vi "QFileDialog.vi"(5 "parent":refnum<class "QWidget.lvclass">, 6 "filter":string, 8 "Error In":errorcluster, 9 "directory":string, 10 "caption":string, 11 "Post-Bundled Subclass":refnum<class "QFileDialog.lvclass">) -> (0 "Error Out":errorcluster, 3 "New QFileDialog":refnum<class "QFileDialog.lvclass">)   [LabVIEW 2014, in "QFileDialog.lvclass"]
doc: "LabVIEW-specific documentation is not yet available. See <b>http://doc.qt.io/qt-5/QFileDialog.html#QFileDialog</b>"
uses:
  QFileDialog.lvclass
  QWidget/QWidget.lvclass
  LQ Core/LQCoreEngine/_Internal/LQIdentity Registry Action.ctl
  LQ Core/LQIdentity/LQIdentity.lvclass/LQIdentity.ctl
  LQ Core/LQCoreEngine/LQCoreEngine.lvclass
  LQ Core/LQ Core.lvlib
  LQ Core/LQIdentity/LQIdentity.lvclass
panel:
  # "Copyright (c) 2016 Sze Howe Koh\n\nThis Source Code Form is subject to the terms of the Mozilla Public\nLicense, v. 2.0. If a copy of the MPL was not distributed with this\nfile, You can obtain one at http://mozilla.org/MPL/2.0/."
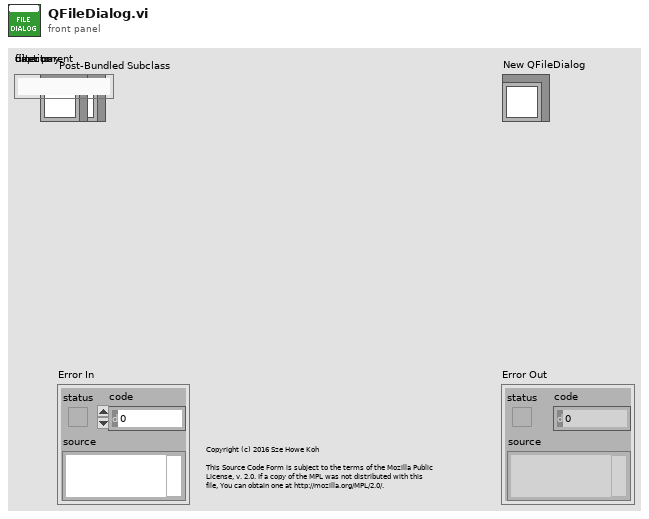
[diagram p1: front panel]
types:
  T1 = typedef "LQ Core.lvlib/LQCoreEngine.lvclass/LQIdentity Registry Action.ctl" = enum16{"Init", "Register LQIdentity", "Get LQIdentity Info", "Deregister LQIdentity"}
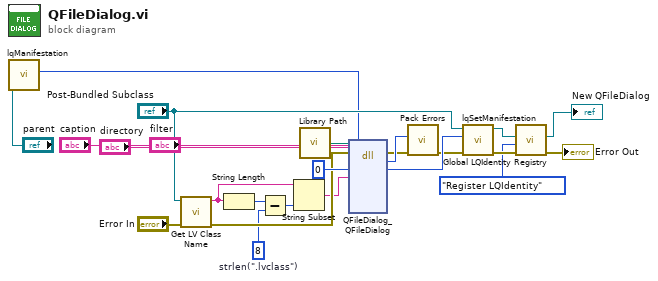
[diagram p0: block diagram]
diagram:
  w9 = 8  # strlen(".lvclass")
  n1 = call "lqManifestation.vi"("LQIdentity in"="parent") -> ("Manifestation"=w4:u64)  [unwired: 9 in, 1 out]
  n2 = call <vilib>:"Get LV Class Name.vi"("error in (no error)"="Error In", "object"="Post-Bundled Subclass") -> ("error out"=w11:errorcluster, "class name"=w7:string)  [unwired: 8 in]
  n3 = String Length(string=w7) -> (length=w10:i32)
  n4 = Subtract(x=w10, y=w9) -> (x-y=w8:i32)
  n5 = String Subset(string=w7, length (rest)=w8) -> (substring=w6:string)  [unwired: 1 in]
  n6 = call "Library Path.vi"() -> ("Library Path"=w22:path)
  n7 = dll-call lib="?" fn="QFileDialog_QFileDialog"(path in=w22, error in=w11, "_retVal"=u64 0 ("_instance"), "_className"=w6, "parent"=w4, "caption"="caption", "directory"="directory", "filter"="filter") -> (error out=w20:errorcluster, w21:i32, "_retVal"=w23:u64)  [unwired: 6 in, 1 out]
  n8 = call "Pack Errors.vi"("Error In"=w20, "Error Code"=w21) -> ("Error Out"=w19:errorcluster)  [unwired: 9 in]
  n9 = call "lqSetManifestation.vi"("Error In"=w19, "Manifestation"=w23, "LQIdentity in"="Post-Bundled Subclass") -> ("Error Out"=w17:errorcluster, "LQIdentity out"=w18:refnum<class "QFileDialog.lvclass">)  [unwired: 7 in]
  n10 = call "Global LQIdentity Registry.vi"("Error In"=w17, "Registry Action"=LQIdentity_Registry_Action."Register LQIdentity", "LQIdentity Info In"=w18) -> ("Error Out"=→"Error Out":errorcluster, "LQIdentity Info Out"=→"New QFileDialog":refnum<class "QFileDialog.lvclass">)  [unwired: 7 in]
